vi "getCenterpt_pel.vi"(4 "markers4":dbl[](array[numeric])) -> (0 "centerxyz":dbl[](array[numeric]))   [LabVIEW 2024]
panel:
  out "Array":i32[](array[numeric])
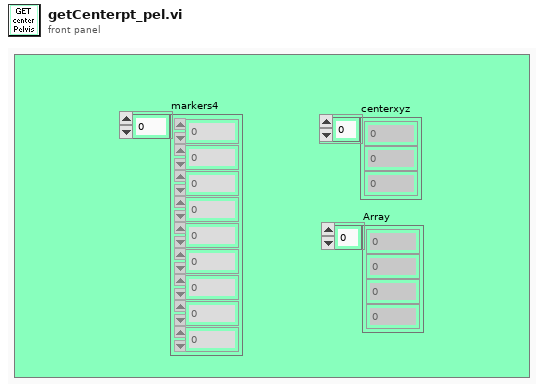
[diagram p1: front panel]
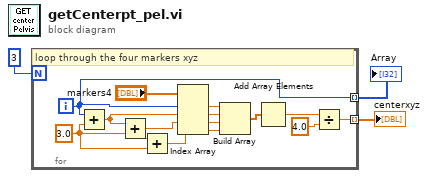
[diagram p0: block diagram]
diagram:
  n1 = for {
    N: 3 -> [_]
    tunnel: [w9] -> w2 mode=indexing
    tunnel: [w4] -> w1 mode=indexing
    i -> [w4]
    w6 = 3.0 ("y")
    # "loop through the four markers xyz"
    n2 = Add(x=w4, y=w6) -> (x+y=w17:dbl)
    n3 = Add(x=w17, y=w6) -> (x+y=w7:dbl)
    n4 = Add(x=w7, y=w6) -> (x+y=w8:dbl)
    n5 = Index Array(array="markers4", index #1=w4, index #2=w17, index #3=w7, index #4=w8) -> (element #1=w15:dbl, element #2=w14:dbl, element #3=w13:dbl, element #4=w5:dbl)
    n6 = Build Array(w15, w14, w13, w5) -> (w12:dbl[])
    n7 = Add Array Elements(numeric array=w12) -> (sum=w11:dbl)
    n8 = Divide(x=w11, y=4.0) -> (x/y=w9:dbl)
  }
  "centerxyz" <- w2
  "Array" <- w1
